vi "PlotScopeData.vi"() -> ()   [LabVIEW 2010]
uses:
  Scope/AddAxisDataConfiguration.vi
  Scope/AddAxisExtendedDataConfiguration.vi
  Motion/EnableSingle.vi
  Scope/StartDataCollectionObsolete.vi
  Motion/MoveIncSingle.vi
  Scope/GetAxisDataResults.vi
  Scope/GetAxisExtendedDataResults.vi
panel:
  in  "axis extended data signal 1":u32(ring)=10 items=["AmplifierPeakCurrent"=303, "AmplifierTemperature"=309, "AnalogInput0"=10, "AnalogInput1"=11, "AnalogInput2"=28, "AnalogInput3"=29, "AnalogOutput0"=36, "AnalogOutput1"=37, "AnalogOutput2"=38, "AnalogOutput3"=39, "AnalogSensorInput"=446, "BoardRevision"=407, "BusVoltage"=375, "BusVoltageNegative"=441, "CapacitanceSensorRawPosition"=415, "CommandOutputType"=389, "ControlEffort"=282, "CurrentCommand"=8, "CurrentFeedback"=7, "DataAcquisitionSamples"=234, "DriveFeedforwardOutput"=404, "DriveMemoryDouble"=42, "DriveMemoryDoublePointer"=206, "DriveMemoryFloat"=41, "DriveMemoryFloatPointer"=205, "DriveMemoryInt16"=157, "DriveMemoryInt16Pointer"=203, "DriveMemoryInt32"=40, "DriveMemoryInt32Pointer"=202, "DriveMemoryInt8"=158, "DriveMemoryInt8Pointer"=204, "DriveTimer"=44, "DriveTimerMax"=319, "DriveTypeID"=305, "EncoderCosine"=27, "EncoderSine"=26, "EnDatAbsolutePosition"=269, "EthernetDebuggingInformation"=365, "FaultPositionFeedback"=372, "FirmwareRevision"=408, "FirmwareVersionBuild"=318, "FirmwareVersionMajor"=315, "FirmwareVersionMinor"=316, "FirmwareVersionPatch"=317, "FPGAVersion"=304, "GalvoLaserOutput"=409, "GalvoLaserPowerCorrectionOutput"=414, "InternalErrorCode"=314, "IOBoardInstalled"=374, "LastTickCounter"=405, "LatchedMarkerPosition"=331, "LoopTransmissionAfter"=31, "LoopTransmissionBefore"=30, "MarkerSearchDistance"=320, "MaximumVoltage"=388, "ModbusBitMasterInputBits"=290, "ModbusBitMasterOutputBits"=291, "ModbusRegDoubleMasterInputWords"=298, "ModbusRegDoubleMasterOutputWords"=299, "ModbusRegInt16MasterInputWords"=292, "ModbusRegInt16MasterOutputWords"=293, "ModbusRegInt32MasterInputWords"=294, "ModbusRegInt32MasterOutputWords"=295, "ModbusRegSingleMasterInputWords"=296, "ModbusRegSingleMasterOutputWords"=297, "MotorCommutationAngle"=373, "MotorTemperature"=447, "MXAbsolutePosition"=311, "NpaqSyncoutStatus"=366, "PhaseACurrentFeedback"=24, "PhaseAVoltageCommand"=300, "PhaseBCurrentFeedback"=25, "PhaseBVoltageCommand"=301, "PhaseCVoltageCommand"=302, "PiezoVoltageCommand"=376, "PiezoVoltageFeedback"=377, "PositionCalibrationGalvo"=419, "PositionCommandDrive"=98, "PositionCommandGalvo"=237, "PositionDetectorVoltage"=235, "PositionFeedbackDrive"=88, "PositionFeedbackGalvo"=327, "ProcessorTemperature"=442, "PSOBitArrayIndex"=310, "PSOCounter1"=229, "PSOCounter2"=230, "PSOCounter3"=231, "PSODistanceArrayIndex"=308, "PSOStatus"=43, "PSOWindow1"=232, "PSOWindow1ArrayIndex"=306, "PSOWindow2"=233, "PSOWindow2ArrayIndex"=307, "ResoluteAbsolutePosition"=369, "ResoluteStatus"=449, "ResolverChannel1"=267, "ResolverChannel2"=268, "ServoUpdateRate"=312, "SettlingTime"=313, "STOStatus"=443, "TemperatureSensor"=332, "TimeSinceReset"=387, "ZHSDifference"=32, "ZHSFiltered"=35, "ZHSSum"=33, "ZHSUnfiltered"=34]
  in  "axis data signal 2":u32(ring) items=["AccelerationCommand"=6, "AccelerationCommandDrive"=181, "AccelerationCommandRaw"=50, "AccelerationCommandRawCal"=193, "AccelerationError"=223, "AccelerationFeedback"=192, "AccelerationMode"=144, "AccelerationRate"=140, "AccelerationTime"=138, "AccelerationType"=142, "AccuracyCorrectionEndingPosition"=418, "AccuracyCorrectionStartingPosition"=417, "AutoFocusError"=410, "AxisFault"=49, "AxisParameter"=76, "AxisStatus"=48, "Backlash"=81, "BacklashTarget"=196, "CalibrationAdjustmentState"=416, "CalibrationAdjustmentValue"=200, "CommunicationRealTimeErrors"=93, "CoordinatedDistanceRemaining"=272, "CoordinatedPositionTarget"=46, "CurrentError"=9, "CurrentFeedbackAverage"=73, "DecelerationMode"=145, "DecelerationRate"=141, "DecelerationTime"=139, "DecelerationType"=143, "DigitalInput"=15, "DigitalOutput"=16, "DistanceLog"=378, "DriveAssert"=453, "DriveCommandsDelayed"=424, "DriveCommandsLost"=425, "DriveCommunicationDelay"=253, "DriveCommunicationDelayLive"=254, "DriveInterfaceCommandCode"=191, "DriveInterfacePacketBit"=261, "DriveInterfacePacketDouble"=189, "DriveInterfacePacketFloat"=190, "DriveInterfacePacketInfoBitValue"=210, "DriveInterfacePacketInt16"=187, "DriveInterfacePacketInt32"=186, "DriveInterfacePacketInt8"=188, "DriveInterfacePacketResponseBit"=262, "DriveInterfacePacketResponseDouble"=259, "DriveInterfacePacketResponseFloat"=260, "DriveInterfacePacketResponseInt16"=257, "DriveInterfacePacketResponseInt32"=256, "DriveInterfacePacketResponseInt8"=258, "DriveInterfacePacketStreamingData"=226, "DriveMotionDelay"=199, "DriveMotionDelayLive"=252, "DriveMotionRate"=198, "DriveSMCMotionState"=168, "DriveStatus"=47, "DriveStatusActual"=99, "FeedforwardCurrent"=208, "FixtureOffset"=18, "FreezeVelocityCommand"=238, "FreezeVelocityFeedback"=239, "GainAffScale"=130, "GainKd1Scale"=333, "GainKiScale"=127, "GainKp1Scale"=334, "GainKpiScale"=129, "GainKposScale"=126, "GainKpScale"=128, "GainVffScale"=131, "GalvoLaserOffDelay"=413, "GalvoLaserOnDelay"=412, "GalvoLaserOutputRaw"=183, "GalvoLaserOutputRawAdvance"=411, "GantryMarkerLatchPosition"=368, "GantryOffset"=91, "GantryRealignState"=100, "HomeState"=82, "InternalPositionOffsets"=241, "JerkCommandRaw"=89, "JogTrajectoryStatus"=116, "MoveReferenceCornerOffset"=359, "MoveReferenceCutterOffset"=358, "MoveReferencePosition"=339, "MoveReferenceTotalOffset"=360, "NormalcyDebug"=84, "PeakCurrent"=78, "PingTest"=117, "PositionCalibration2D"=83, "PositionCalibrationAll"=55, "PositionCalibrationAllDrive"=194, "PositionCommand"=1, "PositionCommandPacket"=163, "PositionCommandRaw"=12, "PositionCommandRawBackwardsDiff"=96, "PositionCommandRawCal"=178, "PositionCommandRawUnfiltered"=227, "PositionCommandRollover"=70, "PositionError"=2, "PositionErrorGalvo"=328, "PositionFeedback"=0, "PositionFeedbackAuxiliary"=14, "PositionFeedbackAuxiliaryRollover"=71, "PositionFeedbackRollover"=69, "PositionOffset"=92, "ProgramPosition"=156, "ProgramPositionCommand"=90, "ProgramPositionFeedback"=107, "ProgramVelocityCommand"=250, "ProgramVelocityFeedback"=251, "SafeZoneState"=323, "ServoRounding"=201, "SpeedTarget"=160, "SpeedTargetActual"=266, "Stability0SettleTime"=86, "Stability1SettleTime"=87, "StatusHighLevelOffsetsLastMsec"=242, "SuppressedFaults"=225, "TotalMoveTime"=85, "TransformAutoOffset"=101, "TransitionOffsetErrors"=228, "VelocityCommand"=4, "VelocityCommandDrive"=180, "VelocityCommandRaw"=13, "VelocityCommandRawBackwardsDiffDelta"=97, "VelocityCommandRawCal"=179, "VelocityError"=5, "VelocityFeedback"=3, "VelocityFeedbackAverage"=72]
  in  "axis data signal 1":u32(ring) items=["AccelerationCommand"=6, "AccelerationCommandDrive"=181, "AccelerationCommandRaw"=50, "AccelerationCommandRawCal"=193, "AccelerationError"=223, "AccelerationFeedback"=192, "AccelerationMode"=144, "AccelerationRate"=140, "AccelerationTime"=138, "AccelerationType"=142, "AccuracyCorrectionEndingPosition"=418, "AccuracyCorrectionStartingPosition"=417, "AutoFocusError"=410, "AxisFault"=49, "AxisParameter"=76, "AxisStatus"=48, "Backlash"=81, "BacklashTarget"=196, "CalibrationAdjustmentState"=416, "CalibrationAdjustmentValue"=200, "CommunicationRealTimeErrors"=93, "CoordinatedDistanceRemaining"=272, "CoordinatedPositionTarget"=46, "CurrentError"=9, "CurrentFeedbackAverage"=73, "DecelerationMode"=145, "DecelerationRate"=141, "DecelerationTime"=139, "DecelerationType"=143, "DigitalInput"=15, "DigitalOutput"=16, "DistanceLog"=378, "DriveAssert"=453, "DriveCommandsDelayed"=424, "DriveCommandsLost"=425, "DriveCommunicationDelay"=253, "DriveCommunicationDelayLive"=254, "DriveInterfaceCommandCode"=191, "DriveInterfacePacketBit"=261, "DriveInterfacePacketDouble"=189, "DriveInterfacePacketFloat"=190, "DriveInterfacePacketInfoBitValue"=210, "DriveInterfacePacketInt16"=187, "DriveInterfacePacketInt32"=186, "DriveInterfacePacketInt8"=188, "DriveInterfacePacketResponseBit"=262, "DriveInterfacePacketResponseDouble"=259, "DriveInterfacePacketResponseFloat"=260, "DriveInterfacePacketResponseInt16"=257, "DriveInterfacePacketResponseInt32"=256, "DriveInterfacePacketResponseInt8"=258, "DriveInterfacePacketStreamingData"=226, "DriveMotionDelay"=199, "DriveMotionDelayLive"=252, "DriveMotionRate"=198, "DriveSMCMotionState"=168, "DriveStatus"=47, "DriveStatusActual"=99, "FeedforwardCurrent"=208, "FixtureOffset"=18, "FreezeVelocityCommand"=238, "FreezeVelocityFeedback"=239, "GainAffScale"=130, "GainKd1Scale"=333, "GainKiScale"=127, "GainKp1Scale"=334, "GainKpiScale"=129, "GainKposScale"=126, "GainKpScale"=128, "GainVffScale"=131, "GalvoLaserOffDelay"=413, "GalvoLaserOnDelay"=412, "GalvoLaserOutputRaw"=183, "GalvoLaserOutputRawAdvance"=411, "GantryMarkerLatchPosition"=368, "GantryOffset"=91, "GantryRealignState"=100, "HomeState"=82, "InternalPositionOffsets"=241, "JerkCommandRaw"=89, "JogTrajectoryStatus"=116, "MoveReferenceCornerOffset"=359, "MoveReferenceCutterOffset"=358, "MoveReferencePosition"=339, "MoveReferenceTotalOffset"=360, "NormalcyDebug"=84, "PeakCurrent"=78, "PingTest"=117, "PositionCalibration2D"=83, "PositionCalibrationAll"=55, "PositionCalibrationAllDrive"=194, "PositionCommand"=1, "PositionCommandPacket"=163, "PositionCommandRaw"=12, "PositionCommandRawBackwardsDiff"=96, "PositionCommandRawCal"=178, "PositionCommandRawUnfiltered"=227, "PositionCommandRollover"=70, "PositionError"=2, "PositionErrorGalvo"=328, "PositionFeedback"=0, "PositionFeedbackAuxiliary"=14, "PositionFeedbackAuxiliaryRollover"=71, "PositionFeedbackRollover"=69, "PositionOffset"=92, "ProgramPosition"=156, "ProgramPositionCommand"=90, "ProgramPositionFeedback"=107, "ProgramVelocityCommand"=250, "ProgramVelocityFeedback"=251, "SafeZoneState"=323, "ServoRounding"=201, "SpeedTarget"=160, "SpeedTargetActual"=266, "Stability0SettleTime"=86, "Stability1SettleTime"=87, "StatusHighLevelOffsetsLastMsec"=242, "STOStatus"=443, "SuppressedFaults"=225, "TotalMoveTime"=85, "TransformAutoOffset"=101, "TransitionOffsetErrors"=228, "VelocityCommand"=4, "VelocityCommandDrive"=180, "VelocityCommandRaw"=13, "VelocityCommandRawBackwardsDiffDelta"=97, "VelocityCommandRawCal"=179, "VelocityError"=5, "VelocityFeedback"=3, "VelocityFeedbackAverage"=72]
  out "Collecting":bool
  in  "taskId":i32(ring)=1 items=["TLibrary", "T01", "T02", "T03", "T04", "T05", "T06", "T07", "T08", "T09", "T10", "T11", "T12", "T13", "T14", "T15", "T16", "T17", "T18", "T19", "T20", "T21", "T22", "T23", "T24", "T25", "T26", "T27", "T28", "T29", "T30", "T31"]
  out "Waveform Chart":waveform(dbl)[](graph)
  in  "points":i32=100 min=1 step=1
  in  "period (ms)":dbl=5.0 min=0.0001 max=1000.0
  in  "move distance":dbl=5.0
  in  "move speed":dbl=25.0
  in  "axisName":string="X"
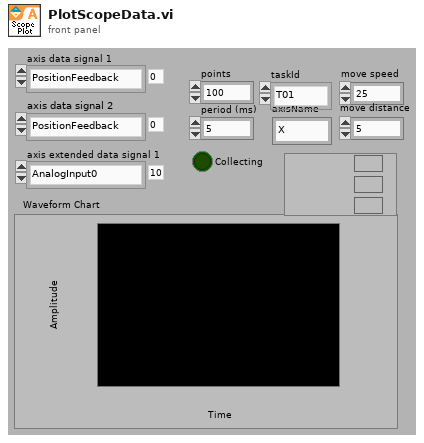
[diagram p1: front panel]
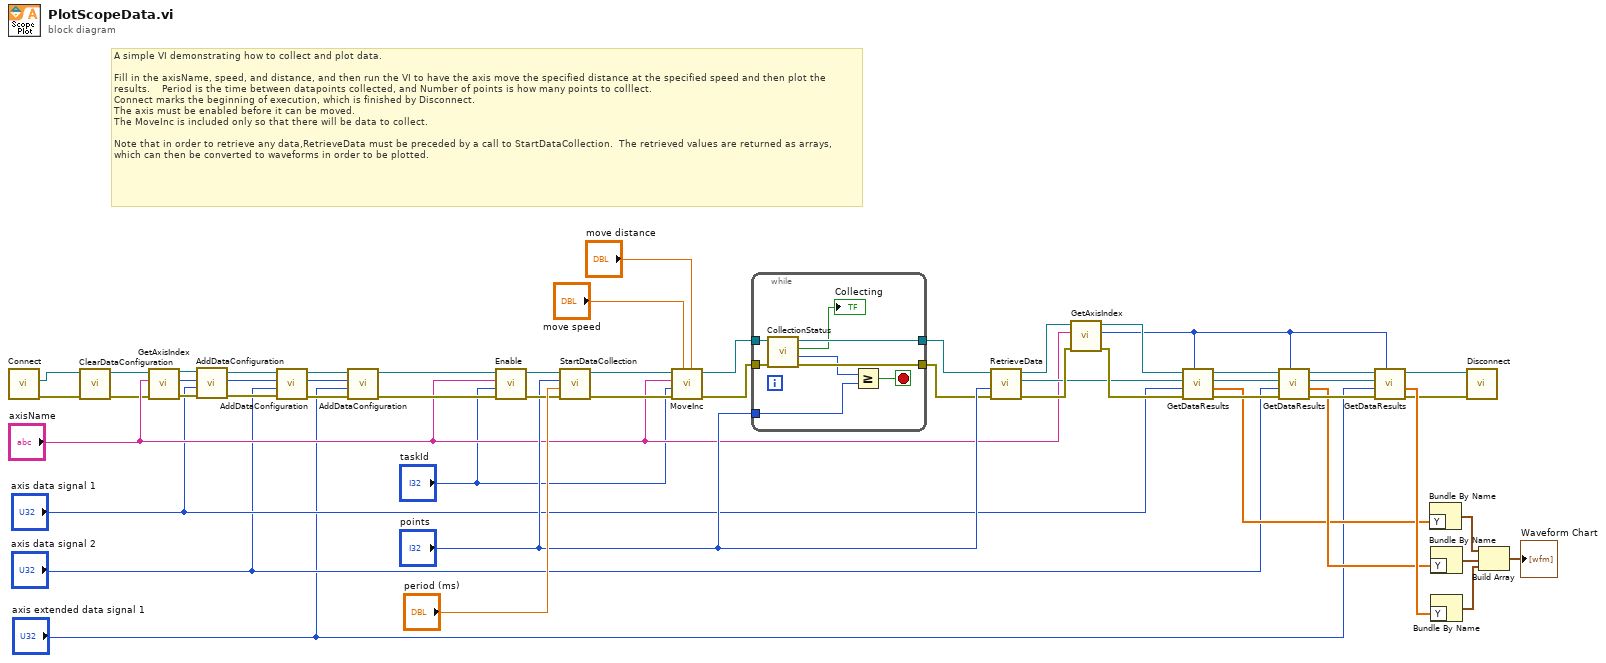
[diagram p0: block diagram]
diagram:
  # "A simple VI demonstrating how to collect and plot data.\n\nFill in the axisName, speed, and distance, and then run the VI to have the axis move the specified distance at the specified speed and then plot the results.    Period is the time between datapoints collected, and Number of points is how many points to colllect.\nConnect marks the beginning of execution, which is finished by Disconnect.\nThe axis must be enabled before it can be moved.\nThe MoveInc is included only so that there will be data to collect.\n\nNote that in order to retrieve any data,RetrieveData must be preceded by a call to StartDataCollection.  The retrieved values are returned as arrays, which can then be converted to waveforms in order to be plotted."
  n1 = call "Connect.vi"() -> ("error out"=w16:errorcluster, "controller"=w18:refnum<k24>)  [unwired: 10 in]
  n2 = call "ClearDataConfiguration.vi"("error in (no error)"=w16, "controller in"=w18) -> ("error out"=w15:errorcluster, "controller out"=w17:refnum<k24>)  [unwired: 8 in]
  n3 = call "GetAxisIndex.vi"("error in (no error)"=w15, "axis name"="axisName", "controller in"=w17) -> ("error out"=w13:errorcluster, "axis index"=w12:i32, "controller out"=w9:refnum<k24>)  [unwired: 6 in]
  n4 = call-poly "AddDataConfiguration.vi"("error in (no error)"=w13, "axis data signal"="axis data signal 1", "axisIndex in"=w12, "controller in"=w9) -> ("error out"=w8:errorcluster, "axisIndex out"=w10:i32, "controller out"=w11:refnum<k24>)  [unwired: 5 in]
  n5 = call-poly "AddDataConfiguration.vi"("error in (no error)"=w8, "axis data signal"="axis data signal 2", "axisIndex in"=w10, "controller in"=w11) -> ("error out"=w36:errorcluster, "axisIndex out"=w33:i32, "controller out"=w37:refnum<k24>)  [unwired: 5 in]
  n6 = call-poly "AddDataConfiguration.vi"("error in (no error)"=w36, "axis extended data signal"="axis extended data signal 1", "axisExtendedIndex in"=w33, "controller in"=w37) -> ("error out"=w35:errorcluster, "controller out"=w34:refnum<k24>)  [unwired: 5 in, 1 out]
  n7 = call-poly "Enable.vi"("error in (no error)"=w35, "taskId"="taskId", "axis name"="axisName", "controller in"=w34) -> ("error out"=w42:errorcluster, "controller out"=w43:refnum<k24>)  [unwired: 6 in]
  n8 = call-poly "StartDataCollection.vi"("error in (no error)"=w42, "Period (msec)"="period (ms)", "Points"="points", "controller in"=w43) -> ("error out"=w41:errorcluster, "controller out"=w44:refnum<k24>)  [unwired: 6 in]
  n9 = call-poly "MoveInc.vi"("distance"="move distance", "speed"="move speed", "error in (no error)"=w41, "taskId"="taskId", "axis name"="axisName", "controller in"=w44) -> ("error out"=w39:errorcluster, "controller out"=w40:refnum<k24>)  [unwired: 4 in]
  n10 = while {
    tunnel: w40 -> [w61]
    tunnel: w39 -> [w60]
    tunnel: "points" -> [w55]
    tunnel: [w58] -> w4
    tunnel: [w57] -> w5
    stop <- w59 stop-if-true
    n11 = call "CollectionStatus.vi"("error in (no error)"=w60, "controller in"=w61) -> ("error out"=w57:errorcluster, "PointsCollected"=w56:i32, "IsCollecting"=→"Collecting":bool, "controller out"=w58:refnum<k24>)  [unwired: 4 in, 2 out]
    n12 = Greater Or Equal?(x=w56, y=w55) -> (x >= y?=w59:bool)
  }
  n13 = call "RetrieveData.vi"("error in (no error)"=w5, "pointsToRetrieve"="points", "controller in"=w4) -> ("error out"=w51:errorcluster, "Data Out"=w26:refnum<k24>, "controller out"=w52:refnum<k24>)  [unwired: 6 in]
  n14 = call "GetAxisIndex.vi"("error in (no error)"=w51, "axis name"="axisName", "controller in"=w52) -> ("error out"=w28:errorcluster, "axis index"=w23:i32, "controller out"=w29:refnum<k24>)  [unwired: 6 in]
  n15 = call-poly "GetDataResults.vi"("axisIndex"=w23, "error in (no error)"=w28, "axis data signal"="axis data signal 1", "Data In"=w26, "controller in"=w29) -> ("error out"=w27:errorcluster, "AxisData"=w20:dbl[], "Data Out"=w25:refnum<k24>, "controller out"=w32:refnum<k24>)  [unwired: 3 in]
  n16 = call-poly "GetDataResults.vi"("axisIndex"=w23, "error in (no error)"=w27, "axis data signal"="axis data signal 2", "Data In"=w25, "controller in"=w32) -> ("error out"=w30:errorcluster, "AxisData"=w21:dbl[], "Data Out"=w24:refnum<k24>, "controller out"=w31:refnum<k24>)  [unwired: 3 in]
  n17 = call-poly "GetDataResults.vi"("axisExtendedIndex"=w23, "error in (no error)"=w30, "axis extended data signal"="axis extended data signal 1", "Data In"=w24, "controller in"=w31) -> ("error out"=w6:errorcluster, "AxisExtendedData"=w22:dbl[], "controller out"=w7:refnum<k24>)  [unwired: 3 in, 1 out]
  n18 = Bundle By Name("Y"=w20) -> (w50:waveform(dbl))  [unwired: 1 in]
  n19 = Bundle By Name("Y"=w21) -> (w49:waveform(dbl))  [unwired: 1 in]
  n20 = Bundle By Name("Y"=w22) -> (w48:waveform(dbl))  [unwired: 1 in]
  n21 = call "Disconnect.vi"("error in (no error)"=w6, "controller"=w7) -> ()  [unwired: 9 in, 1 out]
  n22 = Build Array(w50, w49, w48) -> (→"Waveform Chart":waveform(dbl)[])
